vi "Factorial.vi"(3 "n":i32) -> (1 "n!":dbl format="%.2f")   [LabVIEW 2017, in "NI_Gmath.lvlib"]
doc: "Computes the factorial of <B>n</B>."
uses:
  NI_Gmath.lvlib
  <resource>/lvanlys.dll
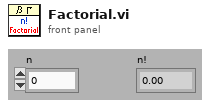
[diagram p1: front panel]
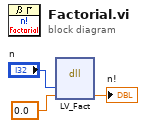
[diagram p0: block diagram]
diagram:
  n1 = dll-call lib="C:/Program Files (x86)/National Instruments/LabVIEW 2017/resource/lvanlys.*" fn="LV_Fact"("n"="n", "n!"=0.0 ("factorial")) -> ("n!"=→"n!":dbl)  [unwired: 5 in, 2 out]
